vi "WriteData (Array of DBL).vi"(6 "value index (0)":u64, 7 "Array of DBL":dbl[](array[numeric]), 8 "error in (no error)":errorcluster, 9 "channel index (0)":u32, 10 "operation (0: create)":T2(ring)=enum."Create", 11 "Excel refnum":T1) -> (0 "error out":errorcluster, 3 "Excel refnum out":T1)   [LabVIEW 2020, in "NI_ExcelFile.lvlib"]
uses:
  <vilib>/express/express shared/NI_ExcelFile/NI_ExcelFile.lvlib
  <vilib>/express/express shared/NI_ExcelFile/Ctrls/ExcelRefnum.ctl
  <vilib>/express/express shared/NI_ExcelFile/Ctrls/MainData.ctl
  <vilib>/express/express shared/NI_ExcelFile/Ctrls/StreamMode.ctl
  <vilib>/express/express shared/NI_ExcelFile/Ctrls/TimeColumnMode.ctl
  <vilib>/express/express shared/NI_ExcelFile/Ctrls/FileAttribute.ctl
  <vilib>/express/express shared/NI_ExcelFile/Ctrls/Columns.ctl
  <vilib>/express/express shared/NI_ExcelFile/Ctrls/ColumnInfo.ctl
  <vilib>/express/express shared/NI_ExcelFile/Ctrls/DataType.ctl
  <vilib>/express/express shared/NI_ExcelFile/Ctrls/wd_recordInfo.ctl
  <vilib>/express/express shared/NI_ExcelFile/Ctrls/disk_TemplateFile.ctl
  <vilib>/express/express shared/NI_ExcelFile/Ctrls/meta_file.ctl
  <vilib>/express/express shared/NI_ExcelFile/Ctrls/meta_Block.ctl
  <vilib>/express/express shared/NI_ExcelFile/Ctrls/meta_BlockType.ctl
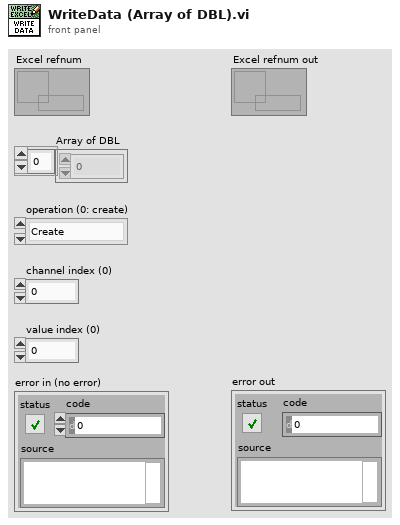
[diagram p1: front panel]
types:
  T1 = typedef "NI_ExcelFile.lvlib/ExcelRefnum.ctl" = refnum<data-value>
  T2 = enum16{"Append values", "Create", "Replace values at index", "Replace all values"}
  T3 = typedef "NI_ExcelFile.lvlib/DataType.ctl" = enum16{"DDT", "WFM", "Array of STR", "Array of DBL", "Array of I8", "Array of I16", "Array of I32", "Array of I64", "Array of SGL", "Array of U8", "Array of U16", "Array of U32", "Array of U64", "Array of Time"}
  T4 = typedef "NI_ExcelFile.lvlib/MainData.ctl" = cluster{"TargetFile":path, "StreamMode":T5, "Append?":bool, "ChunkSize":u64, "TimeColumnMode":T6, "TimestampFormat":string, "AbsoluteTime?":bool, "FileAttribute ":T7, "Column":T8, "FileRef":refnum<k1>, "MemoryRef":refnum<data-value>[], "RecordInfo":T10[], " ChannelPreviousInfo":u32[], "ChannelFirstRecord":u32[], "PredefinedFormattedValueLength":i64, "DiskTemplate":T11}
  T5 = typedef "NI_ExcelFile.lvlib/StreamMode.ctl" = enum16{"File", "Memory"}
  T6 = typedef "NI_ExcelFile.lvlib/TimeColumnMode.ctl" = enum16{"Empty", "OnePerCh", "One"}
  T7 = typedef "NI_ExcelFile.lvlib/FileAttribute.ctl" = cluster{"Creator":string, "Title":string, "SheetName":string}
  T8 = typedef "NI_ExcelFile.lvlib/Columns.ctl" = T9[]
  T9 = typedef "NI_ExcelFile.lvlib/ColumnInfo.ctl" = cluster{"Header":string, "Format":string, "DataType":T3, "Length":u64}
  T10 = typedef "NI_ExcelFile.lvlib/wd_recordInfo.ctl" = cluster{"ChannelIndex":u32, "StartIndex":u64, "Length":u64, "Previous":i32, "Next":i32}
  T11 = typedef "NI_ExcelFile.lvlib/disk_TemplateFile.ctl" = cluster{"XMLRef":refnum<file>[], "ZipPath":path, "MetaFile":T12, "TempFolder":path}
  T12 = typedef "NI_ExcelFile.lvlib/meta_file.ctl" = cluster{"Ref":refnum<file>, "NextRow":i32, "NextPosition":i64, "Block":T13[]}
  T13 = typedef "NI_ExcelFile.lvlib/meta_Block.ctl" = cluster{"Version":u16, "Type":T14, "Length":i32, "Data":string}
  T14 = typedef "NI_ExcelFile.lvlib/meta_BlockType.ctl" = enum16{"NITag", "File", "Column"}
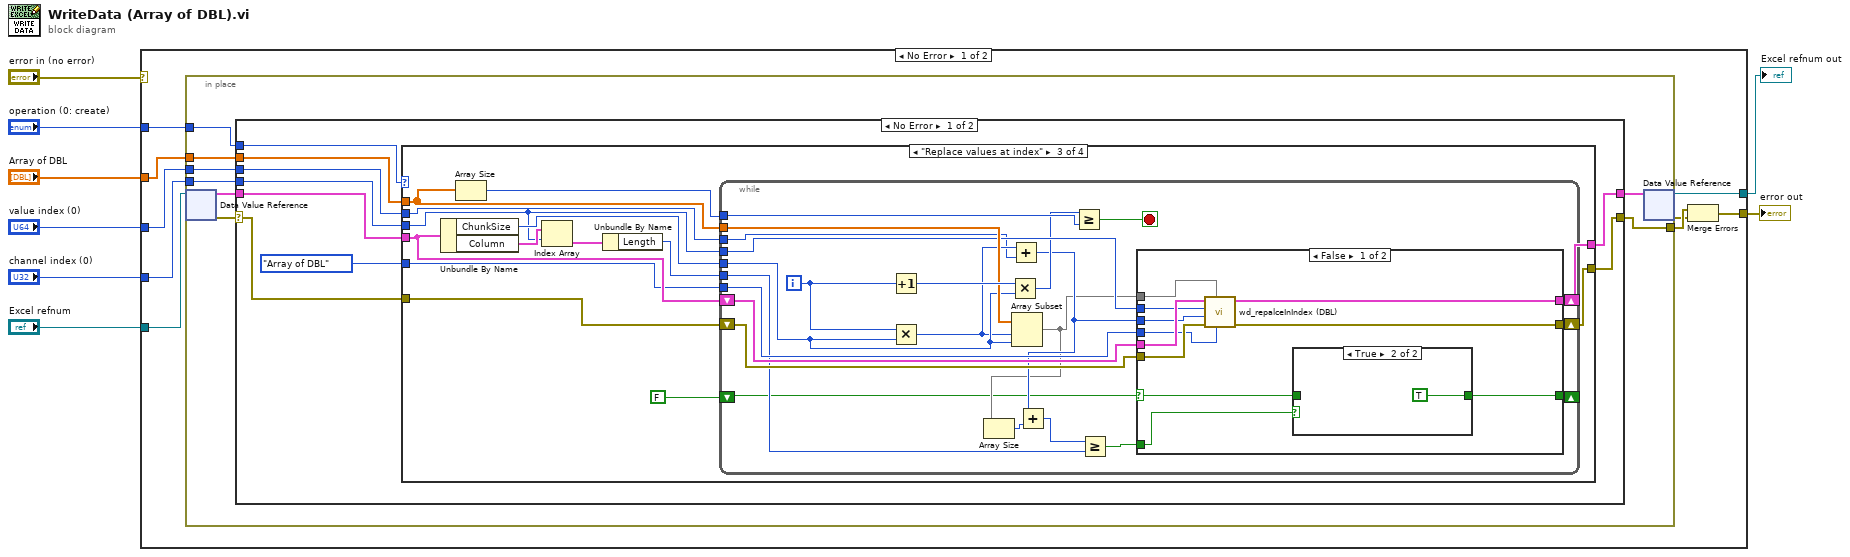
[diagram p0: block diagram]
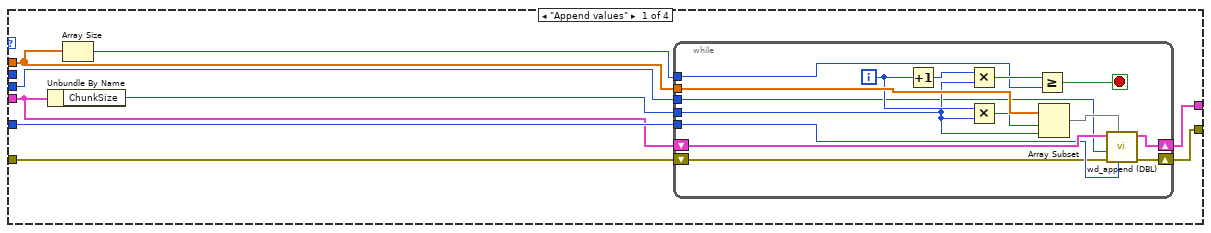
[diagram p2: hidden frame]
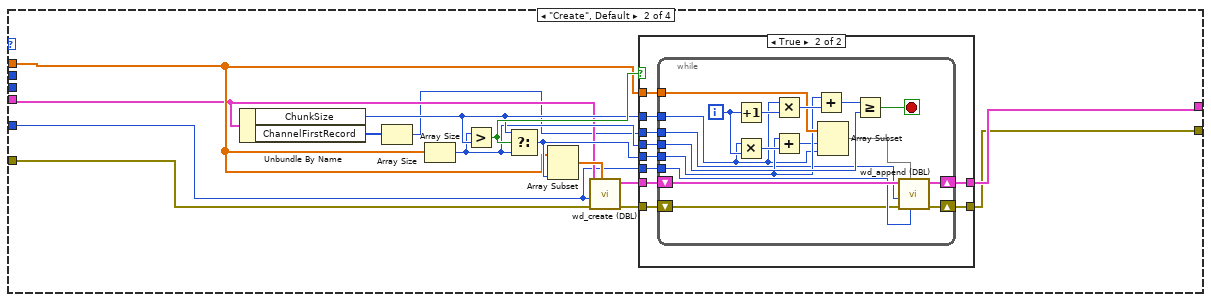
[diagram p3: hidden frame]
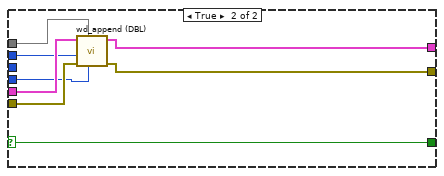
[diagram p6: hidden frame]
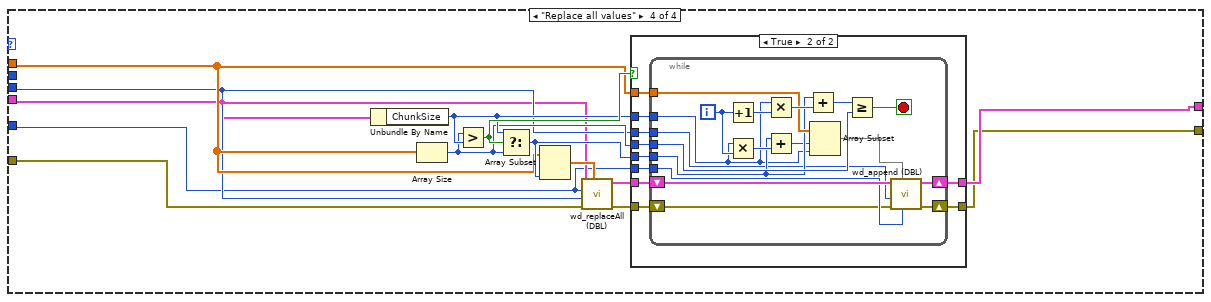
[diagram p7: hidden frame]
diagram:
  n1 = case shown="No Error" "error in (no error)" {
    selector: "error in (no error)" -> [_ w209]
    tunnel: "Array of DBL" -> [w14 _]
    tunnel: [w9 w209] -> w1
    tunnel: "Excel refnum" -> [w17 w208]
    tunnel: [w16 w208] -> w3
    tunnel: "operation (0: create)" -> [w15 _]
    tunnel: "channel index (0)" -> [w13 _]
    tunnel: "value index (0)" -> [w12 _]
    frame No Error {
      n2 = in-place {
        in-place-border: w15 -> [w23]
        in-place-border: w14 -> [w22]
        in-place-border: w13 -> [w21]
        in-place-border: [w20] -> w11
        in-place-border: w12 -> [w19]
        n3 = in-place-dvr #1(w17) -> (w25:T4, w18:errorcluster)
        n4 = case shown="No Error" w18 {
          selector: w18 -> [w26 w206]
          tunnel: w25 -> [w34 w207]
          tunnel: [w33 w207] -> w24
          tunnel: w23 -> [w32 _]
          tunnel: w22 -> [w31 _]
          tunnel: w21 -> [w30 _]
          tunnel: [w29 w206] -> w20
          tunnel: w19 -> [w28 _]
          frame No Error {
            n5 = case shown="\"Replace values at index\"" w32 {
              tunnel: w34 -> [w39 w65 w114 w166]
              tunnel: [w36 w60 w111 w163] -> w33
              tunnel: w31 -> [w42 w66 w115 w168]
              tunnel: w30 -> [w37 _ w108 w167]
              tunnel: w26 -> [w40 w63 w105 w164]
              tunnel: [w35 w59 w110 w162] -> w29
              tunnel: w28 -> [_ _ w112 _]
              tunnel: DataType."Array of DBL" ("new element/subarray") -> [w41 w64 w113 w165]
              frame "Append values" {
                n6 = Unbundle By Name(w39) -> ("ChunkSize"=w38:u64)
                n7 = Array Size(array=w42) -> (size(s)=w43:i32)
                n8 = while {
                  tunnel: w38 -> [w48]
                  tunnel: w43 -> [w56]
                  tunnel: w41 -> [w53]
                  tunnel: w42 -> [w51]
                  shift-right: [w45] -> w36
                  shift-left: w39 -> [w54]
                  shift-right: [w46] -> w35
                  shift-left: w40 -> [w52]
                  tunnel: w37 -> [w44]
                  i -> [w50]
                  stop <- w55 stop-if-true
                  n9 = Increment(x=w50) -> (x+1=w58:i32)
                  n10 = Multiply(x=w58, y=w48) -> (x*y=w57:u64)
                  n11 = Multiply(x=w50, y=w48) -> (x*y=w49:u64)
                  n12 = Greater Or Equal?(x=w57, y=w56) -> (x >= y?=w55:bool)
                  n13 = Array Subset(array=w51, index=w49, length=w48) -> (w47:dbl[])
                  n14 = call <vilib>:"wd_append (DBL).vi"("data type"=w53, "data"=w47, "error in (no error)"=w52, "channel index"=w44, "meta in"=w54) -> ("error out"=w46:errorcluster, "meta out"=w45:T4)  [unwired: 5 in]
                }
              }
              frame "Create", Default {
                n15 = Unbundle By Name(w65) -> ("ChunkSize"=w69:u64, "ChannelFirstRecord"=w62:u32[])
                n16 = Array Size(array=w62) -> (size(s)=w61:i32)
                n17 = Array Size(array=w66) -> (size(s)=w67:i32)
                n18 = Greater?(x=w67, y=w69) -> (0:w72:bool)
                n19 = Select(t=w69, s=w72, f=w67) -> (s? t:f=w68:u64)
                n20 = Array Subset(array=w66, length=w68) -> (w73:dbl[])  [unwired: 1 in]
                n21 = call <vilib>:"wd_create (DBL).vi"("data"=w73, "error in (no error)"=w63, "data type"=w64, "meta in"=w65) -> ("error out"=w70:errorcluster, "meta out"=w71:T4)  [unwired: 6 in]
                n22 = case shown="True" w72 {
                  tunnel: [w75 w77] -> w60
                  tunnel: w71 -> [w75 w81]
                  tunnel: [w74 w76] -> w59
                  tunnel: w70 -> [w74 w78]
                  tunnel: w69 -> [_ w85]
                  tunnel: w68 -> [_ w84]
                  tunnel: w67 -> [_ w83]
                  tunnel: w66 -> [_ w82]
                  tunnel: w61 -> [_ w80]
                  tunnel: w64 -> [_ w79]
                  frame False {
                  }
                  frame True {
                    n23 = while {
                      tunnel: w85 -> [w93]
                      tunnel: w84 -> [w95]
                      tunnel: w83 -> [w100]
                      tunnel: w82 -> [w98]
                      shift-right: [w90] -> w77
                      shift-left: w81 -> [w91]
                      tunnel: w80 -> [w89]
                      tunnel: w79 -> [w88]
                      shift-right: [w86] -> w76
                      shift-left: w78 -> [w87]
                      i -> [w97]
                      stop <- w99 stop-if-true
                      n24 = Increment(x=w97) -> (x+1=w103:i32)
                      n25 = Multiply(x=w93, y=w97) -> (x*y=w96:u64)
                      n26 = Multiply(x=w93, y=w103) -> (x*y=w102:u64)
                      n27 = Add(x=w95, y=w96) -> (x+y=w94:u64)
                      n28 = Add(x=w95, y=w102) -> (x+y=w101:u64)
                      n29 = Array Subset(array=w98, index=w94, length=w93) -> (w92:dbl[])
                      n30 = Greater Or Equal?(x=w101, y=w100) -> (x >= y?=w99:bool)
                      n31 = call <vilib>:"wd_append (DBL).vi"("data type"=w88, "data"=w92, "error in (no error)"=w87, "channel index"=w89, "meta in"=w91) -> ("error out"=w86:errorcluster, "meta out"=w90:T4)  [unwired: 5 in]
                    }
                  }
                }
              }
              frame "Replace values at index" {
                n32 = Unbundle By Name(w114) -> ("ChunkSize"=w116:u64, "Column"=w109:T8)
                n33 = Array Size(array=w115) -> (size(s)=w117:i32)
                n34 = Index Array(array=w109, index=w108) -> (element=w107:T9)
                n35 = Unbundle By Name(w107) -> ("Length"=w106:u64)
                n36 = while {
                  tunnel: w116 -> [w135]
                  tunnel: w117 -> [w139]
                  tunnel: w113 -> [w131]
                  tunnel: w115 -> [w137]
                  shift-right: [w130] -> w111
                  shift-left: w114 -> [w133]
                  shift-right: [w129] -> w110
                  shift-left: w105 -> [w132]
                  tunnel: w108 -> [w134]
                  tunnel: w112 -> [w126]
                  tunnel: w106 -> [w124]
                  shift-right: [w118] -> _
                  shift-left: FALSE ("Append?") -> [w119]
                  i -> [w136]
                  stop <- w138 stop-if-true
                  n37 = Increment(x=w136) -> (x+1=w140:i32)
                  n38 = Multiply(x=w136, y=w135) -> (x*y=w128:u64)
                  n39 = Multiply(x=w140, y=w135) -> (x*y=w127:u64)
                  n40 = Add(x=w128, y=w126) -> (x+y=w122:u64)
                  n41 = Array Subset(array=w137, index=w128, length=w135) -> (w120:dbl[])
                  n42 = Array Size(array=w120) -> (size(s)=w121:i32)
                  n43 = Add(x=w122, y=w121) -> (x+y=w125:u64)
                  n44 = Greater Or Equal?(x=w127, y=w139) -> (x >= y?=w138:bool)
                  n45 = Greater Or Equal?(x=w125, y=w124) -> (x >= y?=w123:bool)
                  n46 = case shown="False" w119 {
                    selector: w119 -> [w142 w154]
                    tunnel: w134 -> [w144 w159]
                    tunnel: w133 -> [w151 w160]
                    tunnel: w120 -> [w150 w161]
                    tunnel: w132 -> [w149 w158]
                    tunnel: w122 -> [w146 _]
                    tunnel: w131 -> [w148 w157]
                    tunnel: [w145 w156] -> w130
                    tunnel: [w147 w155] -> w129
                    tunnel: w123 -> [w143 _]
                    tunnel: [w141 w154] -> w118
                    frame False {
                      n47 = call <vilib>:"wd_repalceInIndex (DBL).vi"("data type"=w148, "data"=w150, "error in (no error)"=w149, "value index"=w146, "channel index"=w144, "meta in"=w151) -> ("error out"=w147:errorcluster, "meta out"=w145:T4)  [unwired: 4 in]
                      n48 = case shown="True" w143 {
                        tunnel: w142 -> [w152 _]
                        tunnel: [w152 TRUE] -> w141
                        frame False {
                        }
                        frame True {
                        }
                      }
                    }
                    frame True {
                      n49 = call <vilib>:"wd_append (DBL).vi"("data type"=w157, "data"=w161, "error in (no error)"=w158, "channel index"=w159, "meta in"=w160) -> ("error out"=w155:errorcluster, "meta out"=w156:T4)  [unwired: 5 in]
                    }
                  }
                }
              }
              frame "Replace all values" {
                n50 = Unbundle By Name(w166) -> ("ChunkSize"=w171:u64)
                n51 = Array Size(array=w168) -> (size(s)=w169:i32)
                n52 = Greater?(x=w169, y=w171) -> (0:w174:bool)
                n53 = Select(t=w171, s=w174, f=w169) -> (s? t:f=w170:u64)
                n54 = Array Subset(array=w168, length=w170) -> (w175:dbl[])  [unwired: 1 in]
                n55 = call <vilib>:"wd_replaceAll (DBL).vi"("data"=w175, "error in (no error)"=w164, "channel index"=w167, "data type"=w165, "meta in"=w166) -> ("error out"=w172:errorcluster, "meta out"=w173:T4)  [unwired: 5 in]
                n56 = case shown="True" w174 {
                  tunnel: [w177 w179] -> w163
                  tunnel: w173 -> [w177 w183]
                  tunnel: [w176 w178] -> w162
                  tunnel: w172 -> [w176 w180]
                  tunnel: w171 -> [_ w187]
                  tunnel: w170 -> [_ w186]
                  tunnel: w169 -> [_ w185]
                  tunnel: w168 -> [_ w184]
                  tunnel: w167 -> [_ w182]
                  tunnel: w165 -> [_ w181]
                  frame False {
                  }
                  frame True {
                    n57 = while {
                      tunnel: w187 -> [w195]
                      tunnel: w186 -> [w197]
                      tunnel: w185 -> [w202]
                      tunnel: w184 -> [w200]
                      shift-right: [w192] -> w179
                      shift-left: w183 -> [w193]
                      tunnel: w182 -> [w191]
                      tunnel: w181 -> [w190]
                      shift-right: [w188] -> w178
                      shift-left: w180 -> [w189]
                      i -> [w199]
                      stop <- w201 stop-if-true
                      n58 = Increment(x=w199) -> (x+1=w205:i32)
                      n59 = Multiply(x=w195, y=w199) -> (x*y=w198:u64)
                      n60 = Multiply(x=w195, y=w205) -> (x*y=w204:u64)
                      n61 = Add(x=w197, y=w198) -> (x+y=w196:u64)
                      n62 = Add(x=w197, y=w204) -> (x+y=w203:u64)
                      n63 = Array Subset(array=w200, index=w196, length=w195) -> (w194:dbl[])
                      n64 = Greater Or Equal?(x=w203, y=w202) -> (x >= y?=w201:bool)
                      n65 = call <vilib>:"wd_append (DBL).vi"("data type"=w190, "data"=w194, "error in (no error)"=w189, "channel index"=w191, "meta in"=w193) -> ("error out"=w188:errorcluster, "meta out"=w192:T4)  [unwired: 5 in]
                    }
                  }
                }
              }
            }
          }
          frame Error {
          }
        }
        n66 = in-place-dvr #1(w24) -> (w16:T1, w10:errorcluster)
      }
      n67 = Merge Errors(w11, w10) -> (w9:errorcluster)
    }
    frame Error {
    }
  }
  "Excel refnum out" <- w3
  "error out" <- w1
